vi "Test if the tree selection gets the correct type.vi"(8 "error in":errorcluster, 11 "TestCase in":refnum<class "Tree Selection.lvclass">) -> (0 "error out":errorcluster, 3 "TestCase out":refnum<class "Tree Selection.lvclass">)   [LabVIEW 2019, in "Tree Selection.lvclass"]
uses:
  Tree Selection.lvclass
  LabVIEW/Panther Dashboard/Panther Dashboard/Panther Dashboard.lvlib
  LabVIEW/Panther Dashboard/Panther Dashboard/Selection Type--enum.ctl
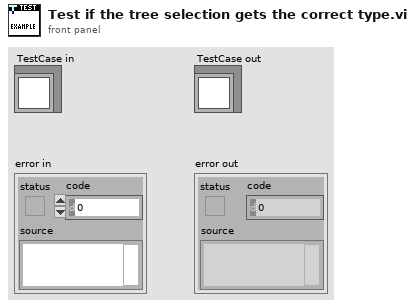
[diagram p1: front panel]
types:
  T1 = typedef "Panther Dashboard.lvlib/Selection Type--enum.ctl" = enum16{"Broadcast", "Request", "Module", "Public API"}
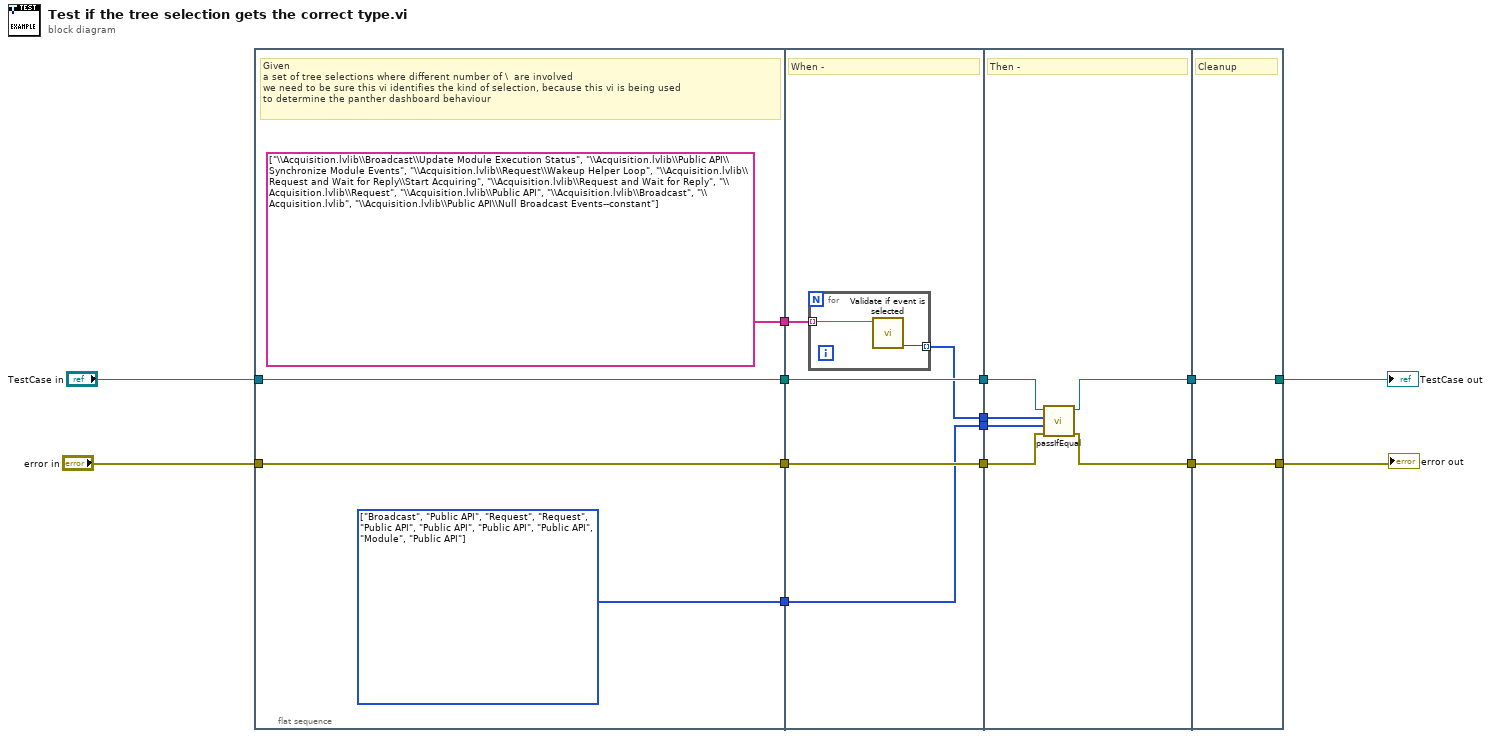
[diagram p0: block diagram]
diagram:
  n1 = flat-sequence {
    tunnel: "error in" -> [w18]
    tunnel: "TestCase in" -> [w17]
    tunnel: [w17] -> w9
    tunnel: [w18] -> w14
    tunnel: [string[] ["\\Acquisition.lvlib\\Broadcast\\Update Module Execution Status", "\\Acquisition.lvlib\\Public API\\Synchronize Module Events", "\\Acquisition.lvlib\\Request\\Wakeup Helper Loop", "\\Acquisition.lvlib\\Request and Wait for Reply\\Start Acquiring", "\\Acquisition.lvlib\\Request and Wait for Reply", "\\Acquisition.lvlib\\Request", "\\Acquisition.lvlib\\Public API", "\\Acquisition.lvlib\\Broadcast", "\\Acquisition.lvlib", "\\Acquisition.lvlib\\Public API\\Null Broadcast Events--constant"]] -> w4
    tunnel: [w15] -> w2
    tunnel: [w22] -> w8
    tunnel: [w23] -> w13
    tunnel: w9 -> [w22]
    tunnel: w14 -> [w23]
    tunnel: w4 -> [w21]
    tunnel: [w20] -> w3
    tunnel: w2 -> [w19]
    tunnel: [w19] -> w1
    tunnel: [w28] -> w7
    tunnel: [w30] -> w12
    tunnel: w8 -> [w29]
    tunnel: w13 -> [w31]
    tunnel: w3 -> [w27]
    tunnel: w1 -> [w26]
    tunnel: [w33] -> w10
    tunnel: [w32] -> w6
    tunnel: w7 -> [w32]
    tunnel: w12 -> [w33]
    frame #0 {
      w15 = T1[] [enum."Broadcast", enum."Public API", enum."Request", enum."Request", enum."Public API", enum."Public API", enum."Public API", enum."Public API", enum."Module", enum."Public API"] items=["Broadcast", "Request", "Module", "Public API"]
      # "Given\na set of tree selections where different number of \\  are involved\nwe need to be sure this vi identifies the kind of selection, because this vi is being used\nto determine the panther dashboard behaviour"
    }
    frame #1 {
      # "When -"
      n2 = for {
        tunnel: w21 -> [w25] mode=indexing
        tunnel: [w24] -> w20 mode=indexing
        n3 = call "Validate if event is selected.vi"("Tree Selection"=w25) -> ("Selection type"=w24:T1)  [unwired: 10 in]
      }
    }
    frame #2 {
      # "Then -"
      n4 = call-dynamic "passIfEqual.vi"("error in (no error)"=w31, "y"=w26, "x"=w27, "TestCase in"=w29) -> ("error out"=w30:errorcluster, "TestCase out"=w28:refnum<class "Tree Selection.lvclass">)  [unwired: 6 in]
    }
    frame #3 {
      # "Cleanup"
    }
  }
  "error out" <- w10
  "TestCase out" <- w6
